vi "Execution.vi"(8 "Error In":errorcluster, 11 "GenAlg_data":T1) -> (0 "Error Out":errorcluster, 3 "GenAlg_data-out":T1)   [LabVIEW 2016]
uses:
  TypeDefs/GenAlg_data.ctl
  TypeDefs/basic_config.ctl
  TypeDefs/element.ctl
  TypeDefs/geration_data.ctl
  TypeDefs/selection_data.ctl
  TypeDefs/SimulatedAnnealing_data.ctl
  TypeDefs/multi_eval_data.ctl
  TypeDefs/termination_data.ctl
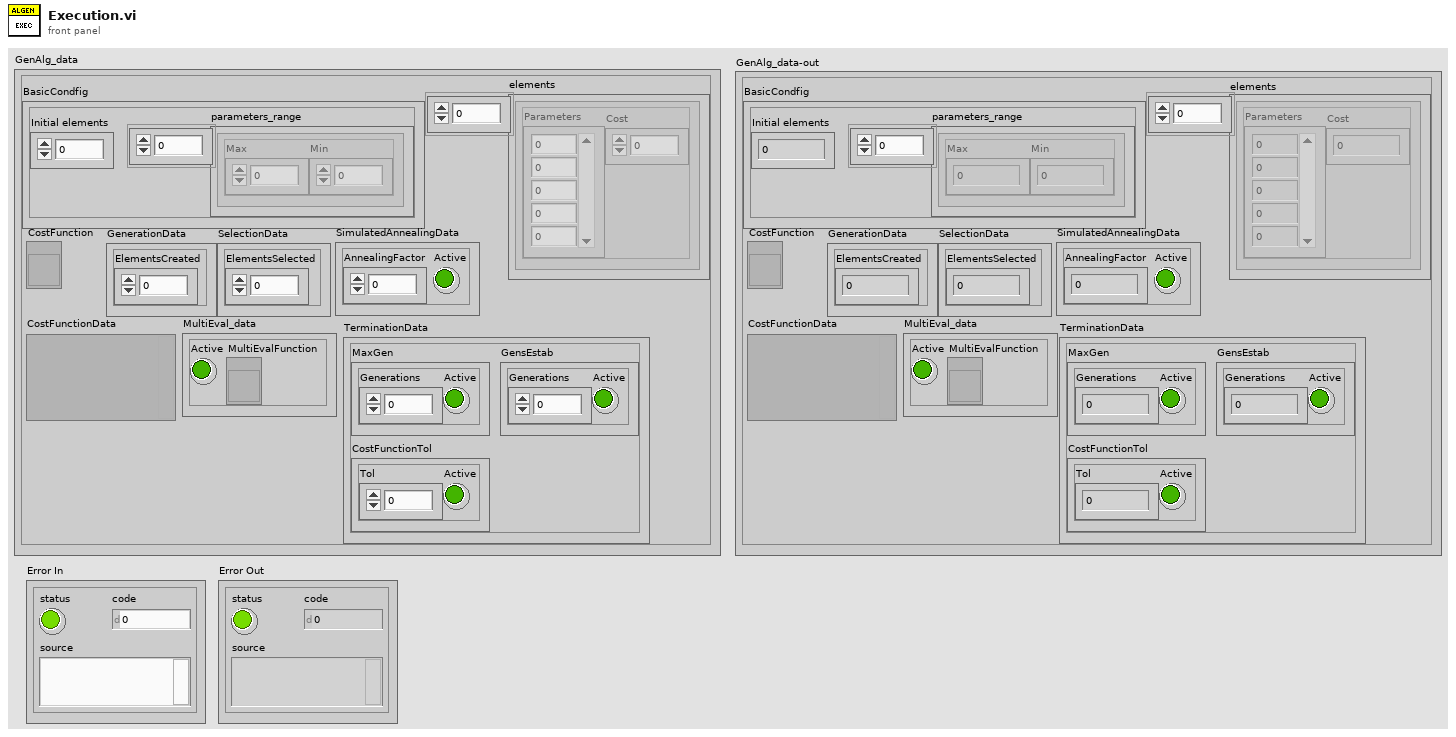
[diagram p1: front panel]
types:
  T1 = typedef "GenAlg_data.ctl" = cluster{"BasicCondfig":T2, "elements":T3[], "CostFunction":refnum<vi>, "GenerationData":T4, "SelectionData":T5, "SimulatedAnnealingData":T6, "CostFunctionData":variant, "MultiEval_data":T7, "TerminationData":T8}
  T2 = typedef "basic_config.ctl" = cluster{"parameters_range":cluster{"Max":dbl, "Min":dbl}[], "Initial elements":i32}
  T3 = typedef "element.ctl" = cluster{"Parameters":dbl[], "Cost":dbl}
  T4 = typedef "geration_data.ctl" = cluster{"ElementsCreated":i32}
  T5 = typedef "selection_data.ctl" = cluster{"ElementsSelected":i32}
  T6 = typedef "SimulatedAnnealing_data.ctl" = cluster{"AnnealingFactor":dbl, "Active":bool}
  T7 = typedef "multi_eval_data.ctl" = cluster{"Active":bool, "MultiEvalFunction":refnum<vi>}
  T8 = typedef "termination_data.ctl" = cluster{"MaxGen":cluster{"Generations":i32, "Active":bool}, "CostFunctionTol":cluster{"Tol":dbl, "Active":bool}, "GensEstab":cluster{"Generations":i32, "Active":bool}}
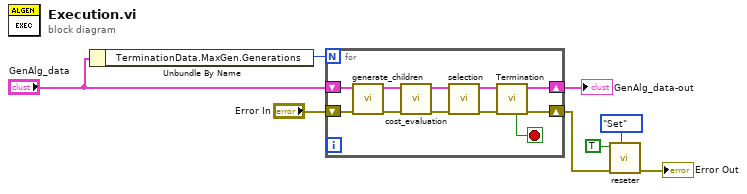
[diagram p0: block diagram]
diagram:
  n1 = Unbundle By Name("GenAlg_data") -> ("TerminationData.MaxGen.Generations"=w6:i32)
  n2 = for {
    N: w6 -> [_]
    shift-right: [w9] -> w2
    shift-left: "Error In" -> [w16]
    shift-right: [w12] -> w5
    shift-left: "GenAlg_data" -> [w19]
    stop <- w10 stop-if-true
    n3 = call "generate_children.vi"("Error In"=w16, "GenAlg_data"=w19) -> ("Error Out"=w17:errorcluster, "GenAlg_data-out"=w18:T1)  [unwired: 8 in]
    n4 = call "cost_evaluation.vi"("Error In"=w17, "GenAlg_data"=w18) -> ("Error Out"=w14:errorcluster, "GenAlg_data-out"=w15:T1)  [unwired: 8 in]
    n5 = call "selection.vi"("Error In"=w14, "GenAlg_data"=w15) -> ("Error Out"=w11:errorcluster, "GenAlg_data-out"=w13:T1)  [unwired: 8 in]
    n6 = call "Termination.vi"("Error In"=w11, "GenAlg_data"=w13) -> ("Error Out"=w9:errorcluster, "GenAlg_data-out"=w12:T1, "Stop"=w10:bool)  [unwired: 7 in]
  }
  "GenAlg_data-out" <- w5
  n7 = call "reseter.vi"("Mode"=enum16{"Init", "Set", "Get"}."Set", "Error In"=w2, "Value"=TRUE) -> ("Error Out"=→"Error Out":errorcluster)  [unwired: 7 in, 1 out]
